vi "JoystickControls.vi"() -> ()   [LabVIEW 2019]
uses:
  TypeDefs/JoystickControl.ctl
panel:
  in  "JoystickControls":T1
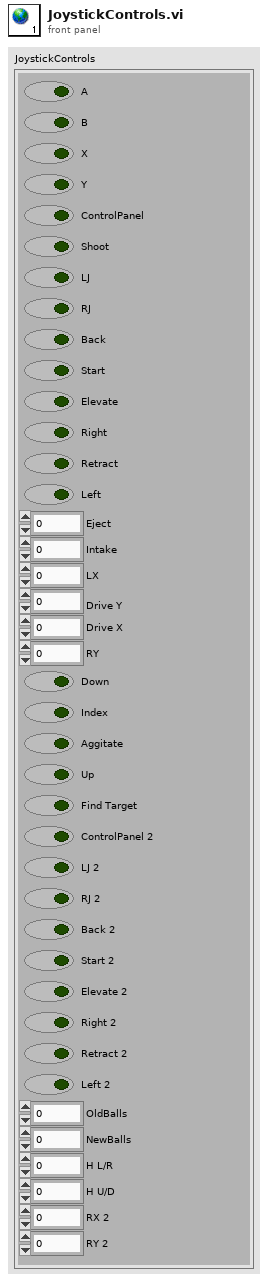
[diagram p1: front panel]
types:
  T1 = typedef "JoystickControl.ctl" = cluster{"A":bool, "B":bool, "X":bool, "Y":bool, "ControlPanel":bool, "Shoot":bool, "LJ":bool, "RJ":bool, "Back":bool, "Start":bool, "Elevate":bool, "Right":bool, "Retract":bool, "Left":bool, "Eject":dbl, "Intake":dbl, "LX":dbl, "Drive Y":dbl, "Drive X":dbl, "RY":dbl, "Down":bool, "Index":bool, "Aggitate":bool, "Up":bool, "Find Target":bool, "ControlPanel 2":bool, "LJ 2":bool, "RJ 2":bool, "Back 2":bool, "Start 2":bool, "Elevate 2":bool, "Right 2":bool, "Retract 2":bool, "Left 2":bool, "OldBalls":dbl, "NewBalls":dbl, "H L/R":dbl, "H U/D":dbl, "RX 2":dbl, "RY 2":dbl}
diagram:
